vi "FindDevice.vi"(8 "error in (no error)":errorcluster, 11 "Multiplexer_Opmux in":refnum<class "Multiplexer_Opmux.lvclass">) -> (0 "error out":errorcluster, 2 "DevFound?":bool, 3 "Multiplexer_Opmux out":refnum<class "Multiplexer_Opmux.lvclass">)   [LabVIEW 2014, in "Multiplexer_Opmux.lvclass"]
uses:
  Multiplexer_Opmux.lvclass
  Multiplexer_Opmux.lvclass/Multiplexer_Opmux.ctl
  <vilib>/Instr/_visa.llb/VISA Configure Serial Port (Instr).vi
  <vilib>/Utility/error.llb/Error Cluster From Error Code.vi
  <vilib>/ErrorRing/Error Ring.xnode
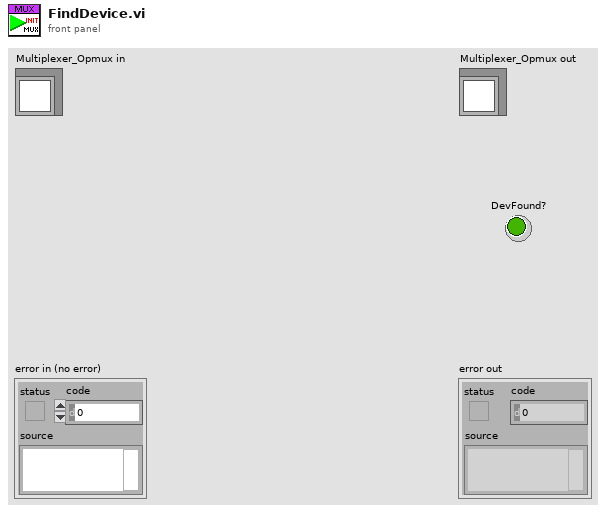
[diagram p1: front panel]
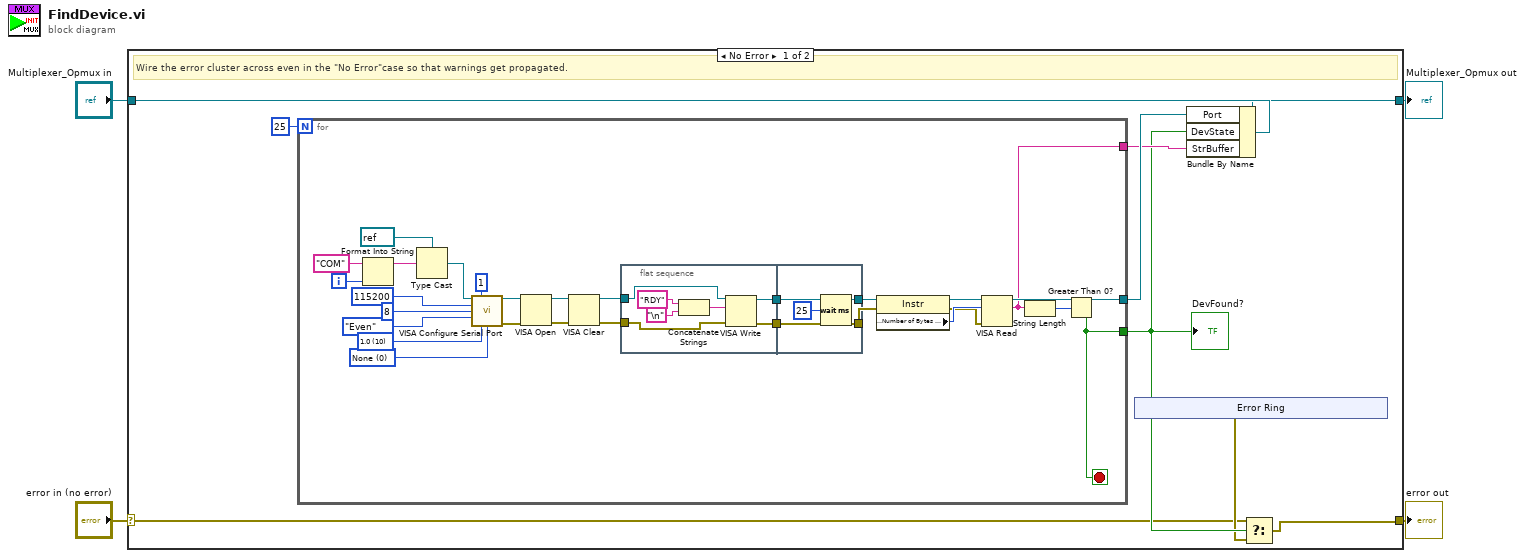
[diagram p0: block diagram]
diagram:
  n1 = case shown="No Error" "error in (no error)" {
    selector: "error in (no error)" -> [w6 w57]
    tunnel: [w5 w57] -> w3
    tunnel: [w12 w56] -> w1
    tunnel: "Multiplexer_Opmux in" -> [w13 w56]
    frame No Error {
      # "Wire the error cluster across even in the \"No Error\"case so that warnings get propagated."
      n2 = for {
        N: 25 -> [_]
        tunnel: [w25] -> w10
        tunnel: [w24] -> w8
        tunnel: [w18] -> w9
        i -> [w20]
        stop <- w24 stop-if-true
        w38 = u16 0 items=["None", "XON/XOFF", "RTS/CTS", "XON/XOFF & RTS/CTS", "DTR/DSR", "XON/XOFF & DTR/DSR"] ("flow control (0:none)")
        w40 = u16 10 items=["1.0"=10, "1.5"=15, "2.0"=20] ("stop bits (10: 1 bit)")
        n3 = Format Into String(initial string="COM", w20) -> (resulting string=w22:string)  [unwired: 2 in, 1 out]
        n4 = Type Cast(type=refnum<visa-resource-name> refnum ("portVisa"), x=w22) -> (*(type *) &x=w19:refnum<visa-resource-name>)
        n5 = call-poly "VISA Configure Serial Port"("VISA resource name"=w19, "timeout (10sec)"=u32 1, "baud rate (9600)"=u32 115200, "data bits (8)"=u16 8, "parity (0:none)"=enum16{"None", "Odd", "Even", "Mark", "Space"}."Even", "stop bits (10: 1 bit)"=w40, "flow control (0:none)"=w38) -> ("VISA resource name out"=w36:refnum<visa-resource-name>, "error out"=w37:errorcluster)  [unwired: 7 in]
        n6 = VISA Open(error in (no error)=w37, VISA resource name=w36) -> (VISA resource name=w34:refnum<visa-resource-name>, error out=w35:errorcluster)  [unwired: 3 in]
        n7 = VISA Clear(VISA resource name=w34, error in (no error)=w35) -> (VISA resource name out=w33:refnum<visa-resource-name>, error out=w32:errorcluster)
        n8 = flat-sequence {
          tunnel: w33 -> [w49]
          tunnel: w32 -> [w48]
          tunnel: [w47] -> w45
          tunnel: [w46] -> w44
          tunnel: [w54] -> w28
          tunnel: [w55] -> w31
          tunnel: w45 -> [w55]
          tunnel: w44 -> [w54]
          frame #0 {
            n9 = Concatenate Strings("RDY", "\n") -> (w50:string)
            n10 = VISA Write(VISA resource name=w49, write buffer=w50, error in (no error)=w48) -> (VISA resource name out=w47:refnum<visa-resource-name>, error out=w46:errorcluster)  [unwired: 1 out]
          }
          frame #1 {
            n11 = Wait (ms)(milliseconds to wait=u32 25) -> ()  [unwired: 1 out]
          }
        }
        n12 = property class="Instr"(reference=w31, error in=w28) -> (reference out=w30:refnum<visa-resource-name>, error out=w27:errorcluster, "Serial Settings:Number of Bytes at Serial Port"=w29:u32)
        n13 = VISA Read(VISA resource name=w30, byte count=w29, error in (no error)=w27) -> (VISA resource name out=w25:refnum<visa-resource-name>, read buffer=w18:string)  [unwired: 2 out]
        n14 = String Length(string=w18) -> (length=w26:i32)
        n15 = Greater Than 0?(x=w26) -> (x > 0?=w24:bool)
      }
      "DevFound?" <- w8
      n16 = xnode "Error Ring"() -> ("error out"=w7:errorcluster)
      n17 = Bundle By Name(cluster=w13, "Port"=w10, "DevState"=w8, "StrBuffer"=w9) -> (w12:refnum<class "Multiplexer_Opmux.lvclass">)
      n18 = Select(t=w6, s=w8, f=w7) -> (s? t:f=w5:errorcluster)
    }
    frame Error {
    }
  }
  "error out" <- w3
  "Multiplexer_Opmux out" <- w1
